vi "_getViExecutionInfo.vi"(8 "error in (no error)":errorcluster, 11 "VI in":refnum<vi>) -> (0 "error out":errorcluster, 2 "VI Execution Info":T1, 3 "VI out":refnum<vi>)   [LabVIEW 2017]
doc: "Returns the execution information for the specified VI reference."
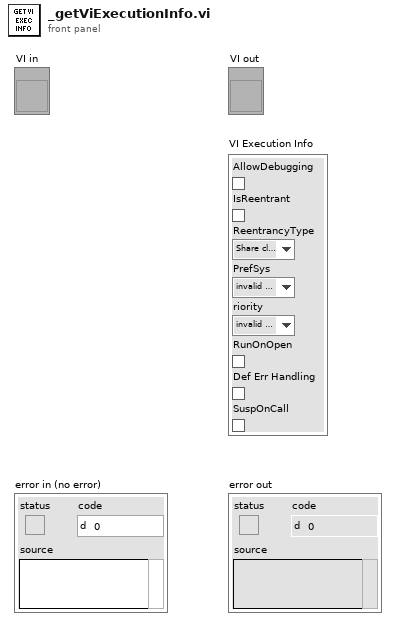
[diagram p1: front panel]
types:
  T1 = cluster{"AllowDebugging":bool, "IsReentrant":bool, "ReentrancyType":enum16{"Share clones between instances", "Preallocate clone for each instance"}, "PrefSys":enum32{"invalid execution system", "user interface", "standard", "instrument i/o", "data acquisition", "other 1", "other 2", "same as caller"}, "riority":enum32{"invalid priority", "background priority", "normal priority", "above normal priority", "high priority", "time critical priority", "subroutine"}, "RunOnOpen":bool, "Def Err Handling":bool, "SuspOnCall":bool}
  T2 = enum16{"Share clones between instances", "Preallocate clone for each instance"}
  T3 = enum32{"invalid execution system", "user interface", "standard", "instrument i/o", "data acquisition", "other 1", "other 2", "same as caller"}
  T4 = enum32{"invalid priority", "background priority", "normal priority", "above normal priority", "high priority", "time critical priority", "subroutine"}
  T5 = cluster{"Exec.AllowDebug":bool, "Exec.IsReentrant":bool, "Exec.ReentrancyType":enum16{"Share clones between instances", "Preallocate clone for each instance"}, "Exec.PrefSys":enum32{"invalid execution system", "user interface", "standard", "instrument i/o", "data acquisition", "other 1", "other 2", "same as caller"}, "Exec.Priority":enum32{"invalid priority", "background priority", "normal priority", "above normal priority", "high priority", "time critical priority", "subroutine"}, "Exec.RunOnOpen":bool, "Def Err Handling":bool, "Exec.SuspOnCall":bool}
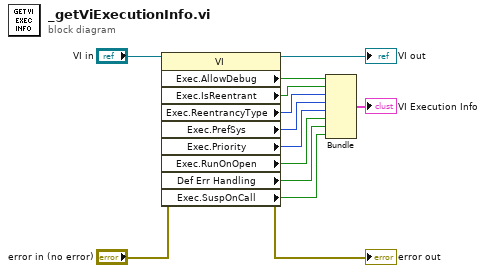
[diagram p0: block diagram]
diagram:
  n1 = property class="VI"(reference="VI in", error in="error in (no error)") -> (reference out=→"VI out":refnum<vi>, error out=→"error out":errorcluster, "Exec.AllowDebug"=w9:bool, "Exec.IsReentrant"=w8:bool, "Exec.ReentrancyType"=w7:T2, "Exec.PrefSys"=w6:T3, "Exec.Priority"=w5:T4, "Exec.RunOnOpen"=w4:bool, "Def Err Handling"=w3:bool, "Exec.SuspOnCall"=w2:bool)
  n2 = Bundle("Exec.AllowDebug"=w9, "Exec.IsReentrant"=w8, "Exec.ReentrancyType"=w7, "Exec.PrefSys"=w6, "Exec.Priority"=w5, "Exec.RunOnOpen"=w4, "Def Err Handling"=w3, "Exec.SuspOnCall"=w2) -> (→"VI Execution Info":T5)  [unwired: 1 in]
